vi "PID1_v1.vi"() -> ()   [LabVIEW 2019]
doc: "Manually blink and LED attached to a digital output channel of a LINX device by clicking and LED control in LabVIEW."
uses:
  <vilib>/addons/control/pid/NI_PID_pid.lvlib
  <vilib>/addons/control/pid/pid.llb/PID Advanced (DBL).vi
  <vilib>/addons/control/pid/pid.llb/PID Structure Conversion (DBL).vi
  <vilib>/addons/control/pid/pid.llb/PID Structure.ctl
  <vilib>/addons/control/pid/pid.llb/PID Time Unit.ctl
  <vilib>/addons/control/pid/pid.llb/PID Gain Unit.ctl
panel:
  out "servo":dbl
  in  "Distance":dbl
  out "Slide":dbl(slide) scale=0.0..60.0
  in  "PID (dt)":dbl
  out "PID (dt)":dbl
  in  "Proportional Unit":T1 items=["Gain (Kc)", "Band (PB)"]
  in  "Derivative Unit":T2 items=["min", "s"]
  in  "Integral Unit":T2 items=["min", "s"]
  in  "PID Topology":T3 items=["Academic (Standard)", "Parallel", "Series"]
  in  "Derivative":dbl format="%#.3g"
  in  "Integral":dbl=0.008 format="%#.3g"
  in  "Proportional":dbl=5.0 format="%#.10f"
  in  "Initialize":bool
  out "Waveform Chart":cluster{"Setpoint":dbl, dbl, "servo":dbl}(graph)
  in  "setpoint range":cluster{"setpoint high":dbl, "setpoint low":dbl}={"setpoint high"=60.0, "setpoint low"=0.0} {"setpoint high" min=0.0 max=60.0 format="%.2f"; "setpoint low" min=0.0 max=60.0 format="%.2f"}
  out "Lamp":bool
  out "output":dbl format="%.1f"
  in  "output range":cluster{"output high":dbl, "output low":dbl}={"output high"=100.0, "output low"=0.0} {"output low" min=0.0 max=2500.0 format="%.2f"; "output high" min=0.0 max=2500.0 format="%.2f"}
  out "Winkel":dbl format="%.1g"
  in  "Setpoint":dbl
  in  "Manual":bool
  in  "Manual setpoint":dbl(slide) scale=0.0..100.0
  in  "Stop Button":bool
  # "Within 1 cm of S.P.\nPID Gain"
  # "Working variable values:"
  # "Distance"
  # "Manual override servo"
  # "PID output\nPID Gain"
  # "PID (dt)                  = 0.02\n\nAveraging distance = 10\n\nAveraging servo       = 10\n\nOutput high            = 70,0\nOutput low              = 0,00\n\nSetpoint high           = 60,0\nSetpoint low            = 0,0\n\nProportional             = 1,0\nIntegral                   = 1,3s\nDerivative               = 1,51s"
  # "Graph\nPID Gain"
  # "Setpoint"
  # "Output range\nPID Gain"
  # "-\nPID Gain"
  # "Setpoint range\nSetpoint range\nPID Gain"
  # "RIO2000"
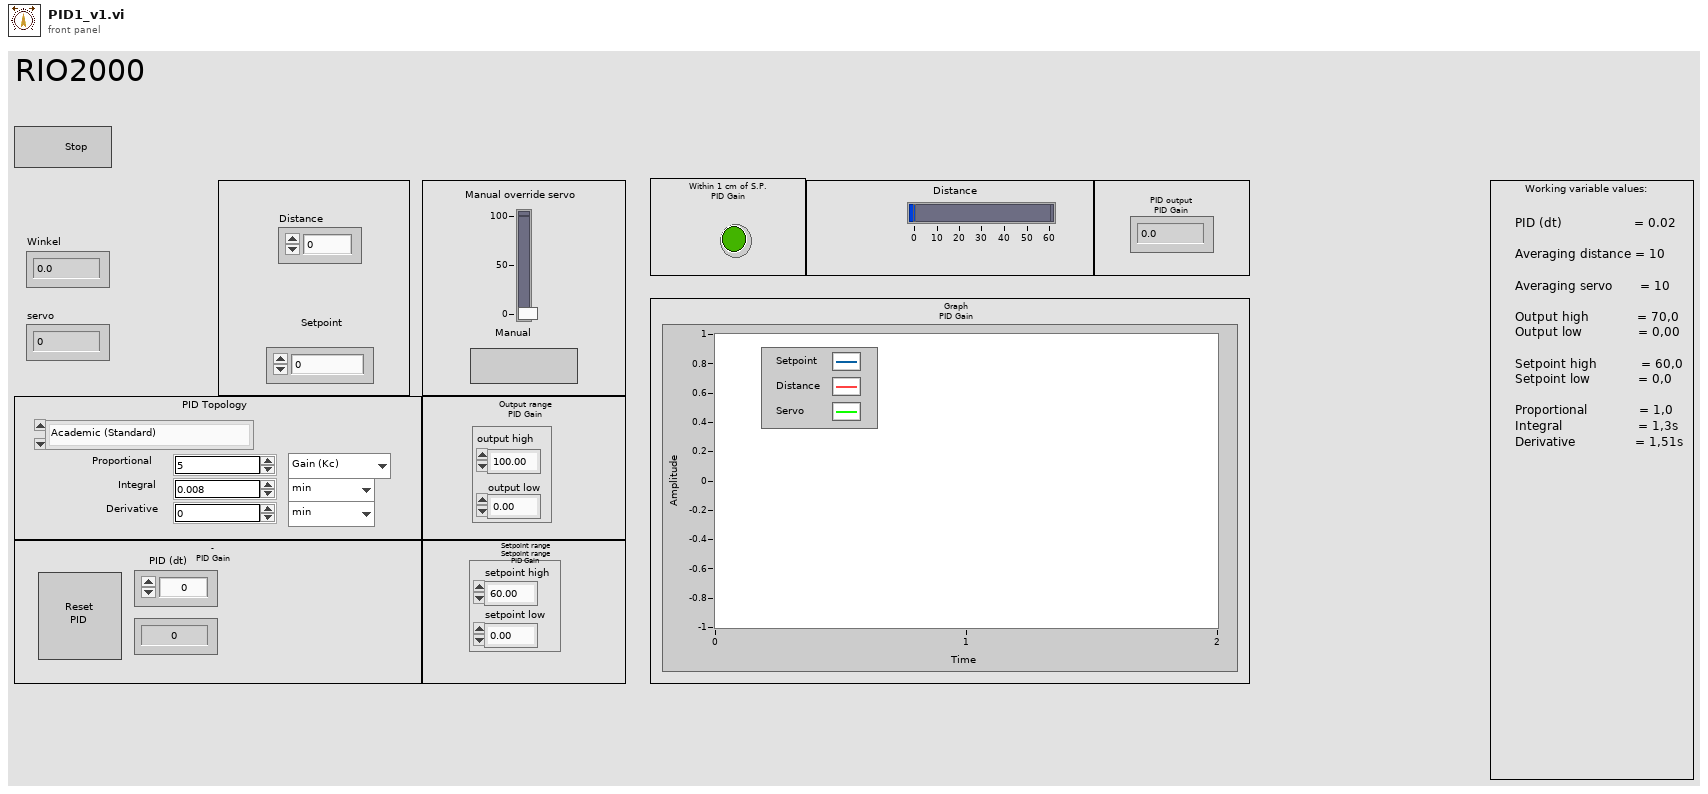
[diagram p1: front panel]
types:
  T1 = typedef "NI_PID_pid.lvlib/PID Gain Unit.ctl" = u16
  T2 = typedef "NI_PID_pid.lvlib/PID Time Unit.ctl" = u16
  T3 = typedef "NI_PID_pid.lvlib/PID Structure.ctl" = u16
  T4 = cluster{"proportional gain (Kc)":dbl, "integral time (Ti, min)":dbl, "derivative time (Td, min)":dbl}
  T5 = cluster{"Setpoint":dbl, "Distance":dbl, "servo":dbl}
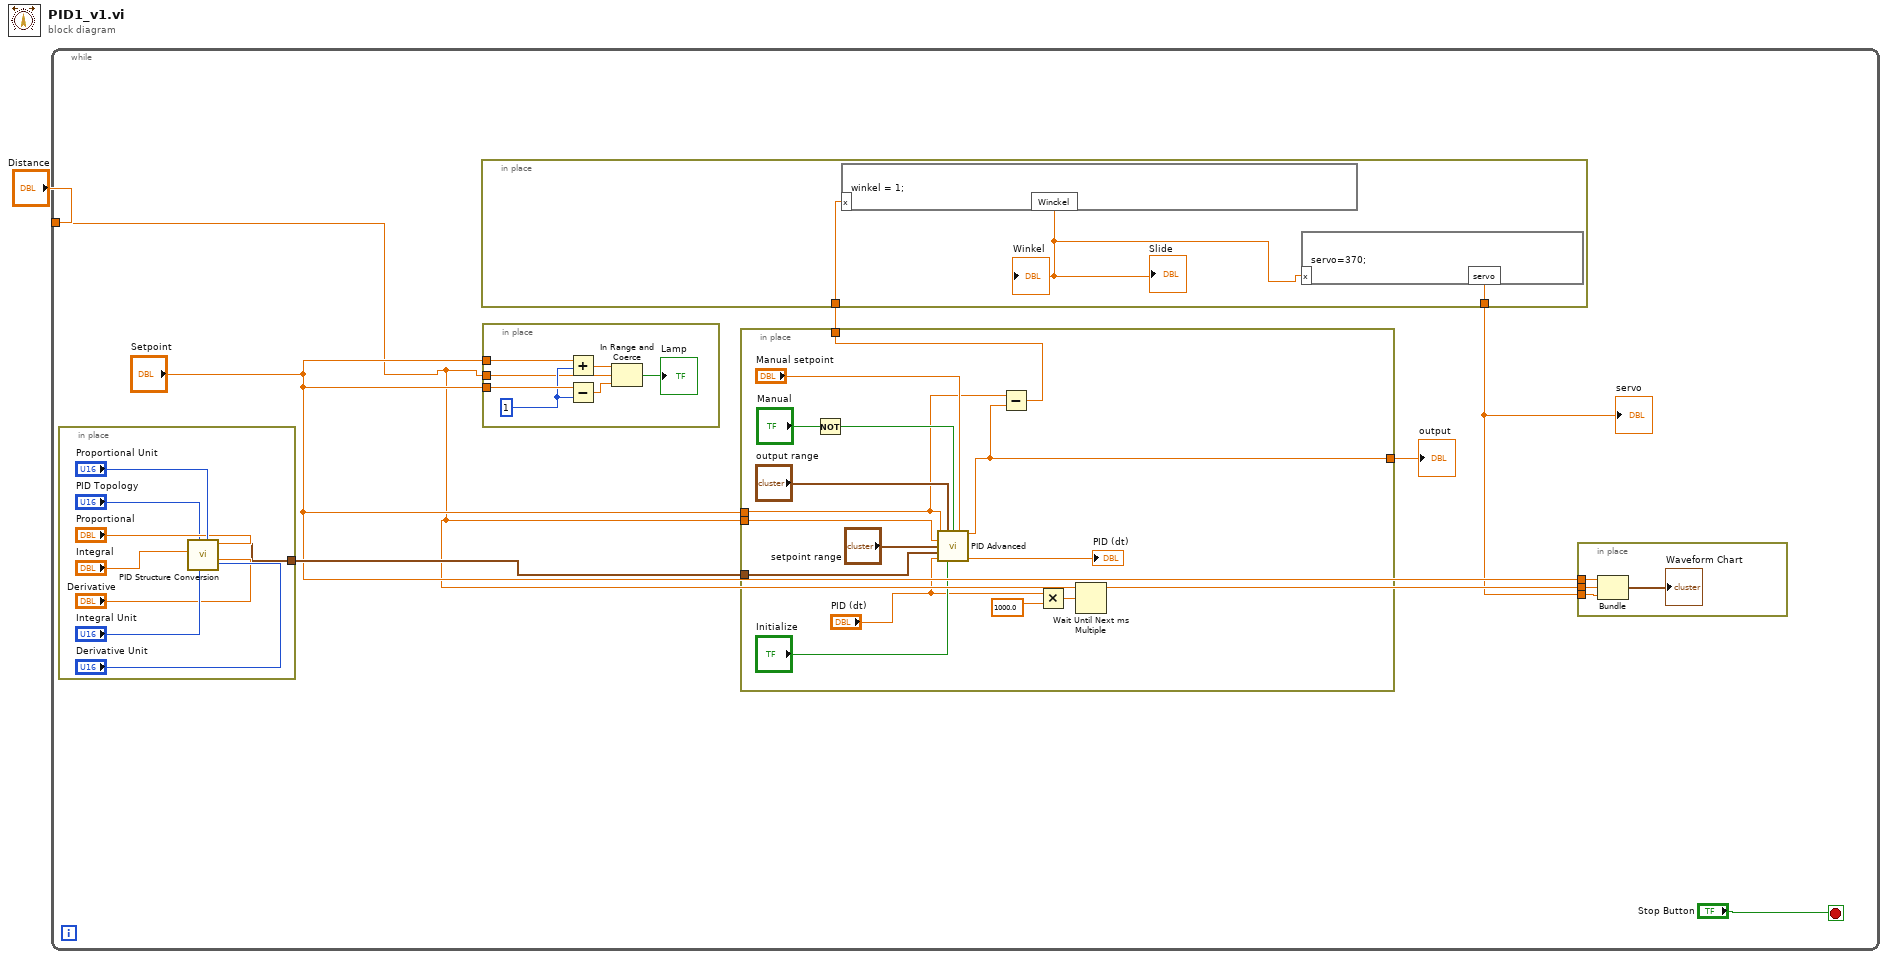
[diagram p0: block diagram]
diagram:
  # "4."
  # "3."
  n1 = while {
    tunnel: "Distance" -> [w6]
    stop <- "Stop Button" stop-if-true
    n2 = in-place {
      in-place-border: [w28] -> w8
      n3 = call-poly <vilib>:"PID Structure Conversion.vi"("derivative unit"="Derivative Unit", "proportional unit"="Proportional Unit", "integral unit"="Integral Unit", "PID structure"="PID Topology", "derivative"="Derivative", "integral"="Integral", "proportional"="Proportional") -> ("PID gains"=w28:T4)  [unwired: 4 in]
    }
    n4 = in-place {
      in-place-border: "Setpoint" -> [w43]
      in-place-border: "Setpoint" -> [w42]
      in-place-border: w6 -> [w39]
      w41 = 1
      n5 = Add(x=w42, y=w41) -> (x+y=w45:dbl)
      n6 = Subtract(x=w43, y=w41) -> (x-y=w40:dbl)
      n7 = In Range and Coerce(upper limit=w45, x=w39, lower limit=w40) -> (In Range?=→"Lamp":bool)  [unwired: 1 out]
    }
    n8 = in-place {
      in-place-border: w8 -> [w21]
      in-place-border: "Setpoint" -> [w14]
      in-place-border: w6 -> [w18]
      in-place-border: [w15] -> w5
      in-place-border: [w13] -> w4
      n9 = Not(x="Manual") -> (.not. x?=w23:bool)
      n10 = call-poly <vilib>:"PID Advanced.vi"("setpoint"=w14, "output range"="output range", "auto? (T)"=w23, "manual control"="Manual setpoint", "process variable"=w18, "setpoint range"="setpoint range", "PID gains"=w21, "dt (s)"="PID (dt)", "reinitialize? (F)"="Initialize") -> ("output"=w15:dbl, "dt out (s)"=→"PID (dt)":dbl)  [unwired: 5 in]
      n11 = Subtract(x=w14, y=w15) -> (x-y=w13:dbl)
      n12 = Multiply(x="PID (dt)", y=1000.0) -> (x*y=w19:dbl)
      n13 = Wait Until Next ms Multiple(millisecond multiple=w19) -> ()  [unwired: 1 out]
    }
    "output" <- w5
    n14 = in-place {
      in-place-border: w4 -> [w38]
      in-place-border: [w36] -> w3
      n15 = formula code="winkel = 1;"("x"=w38) -> ("Winckel"=w37:dbl)
      "Winkel" <- w37
      "Slide" <- w37
      n16 = formula code="servo=370;"("x"=w37) -> ("servo"=w36:dbl)
    }
    "servo" <- w3
    n17 = in-place {
      in-place-border: "Setpoint" -> [w11]
      in-place-border: w6 -> [w10]
      in-place-border: w3 -> [w9]
      n18 = Bundle("Setpoint"=w11, "Distance"=w10, "servo"=w9) -> (→"Waveform Chart":T5)  [unwired: 1 in]
    }
  }
